vi "数据导入工具-main.vi"() -> ()   [LabVIEW 2016]
uses:
  <vilib>/Utility/sysdir.llb/System Directory Type.ctl
  <vilib>/addons/database/Connection.llb/DB Tools Open Connec (String).vi
  <userlib>/_LVST/sqlite_api/Core/Tables/SQLite_List Tables.vi
  <vilib>/addons/database/NI_Database_API.lvlib
  Access/Access Lib.lvlib
panel:
  in  "Password":string
  in  "Sqlite加密":bool
  in  "Sqlite解密":bool
  out "selected path":path caption="所选路径"
  in  "导入日志":string
  in  "导入SQLite":bool
  in  "ACCESS数据表":bool
  in  "列表框":i32[](listbox)
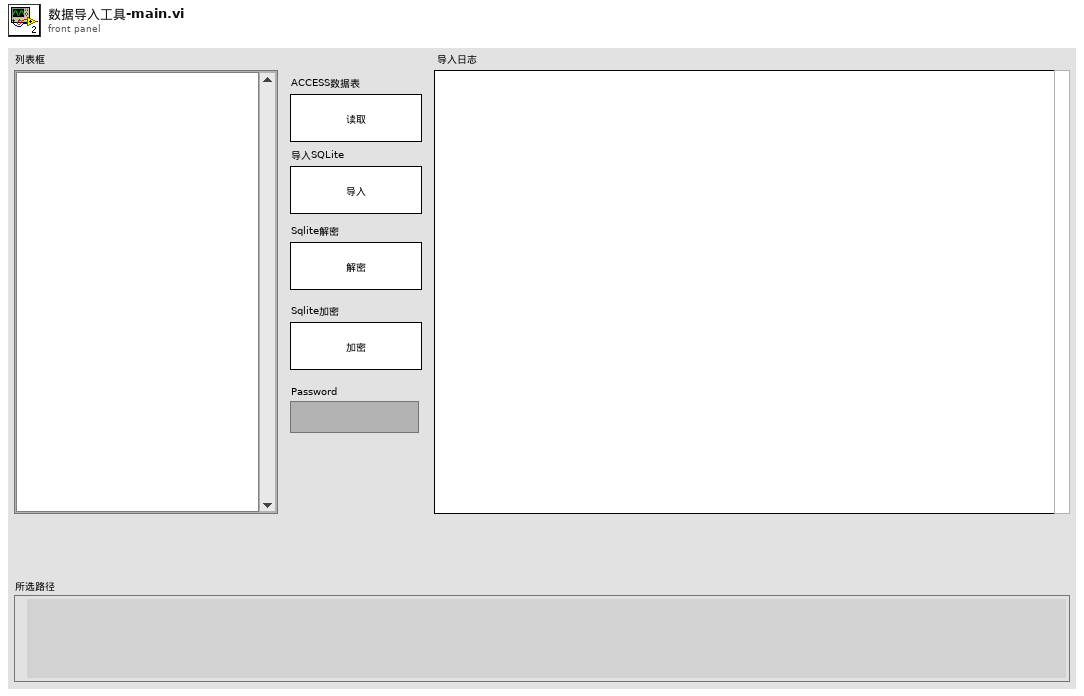
[diagram p1: front panel]
types:
  T1 = typedef "System Directory Type.ctl" = i32
  T2 = typedef "NI_Database_API.lvlib/Conn ObjectReference.ctl" = refnum<k1>
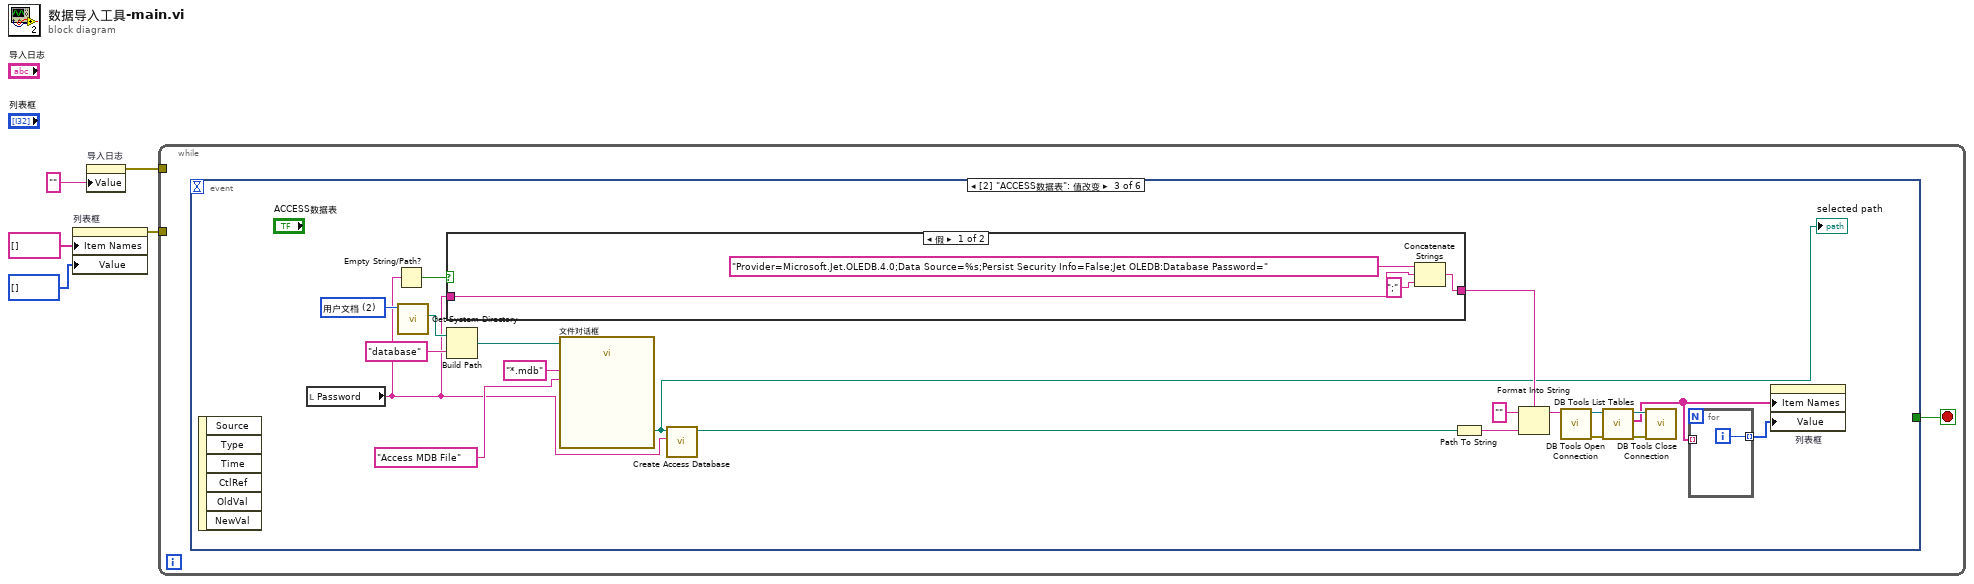
[diagram p0: block diagram]
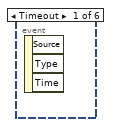
[diagram p2: hidden frame]
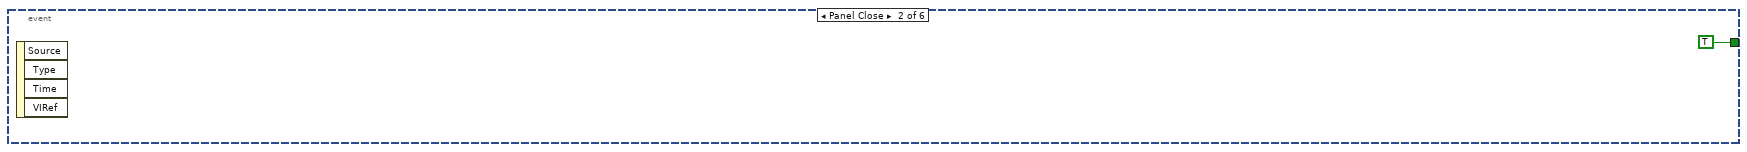
[diagram p3: hidden frame]
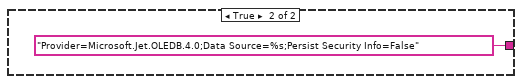
[diagram p4: hidden frame]
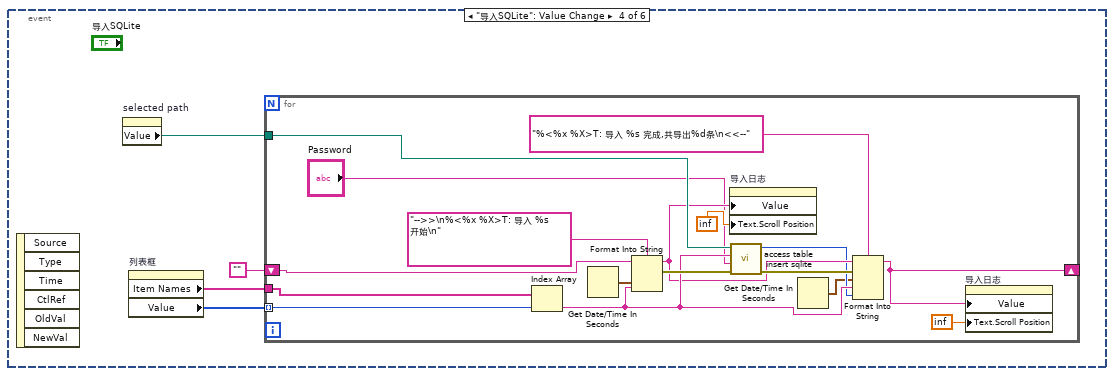
[diagram p5: hidden frame]
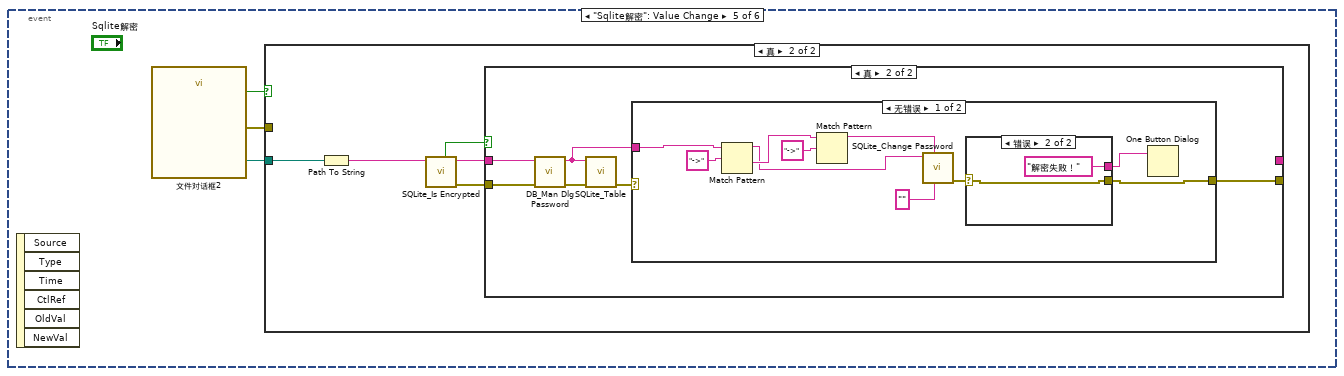
[diagram p6: hidden frame]
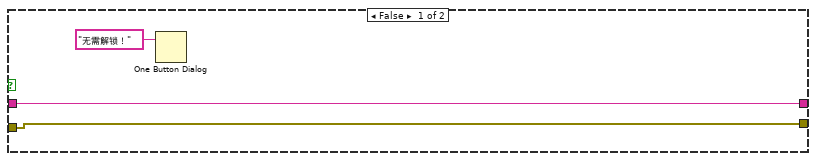
[diagram p8: hidden frame]
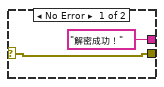
[diagram p9: hidden frame]
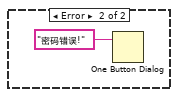
[diagram p10: hidden frame]
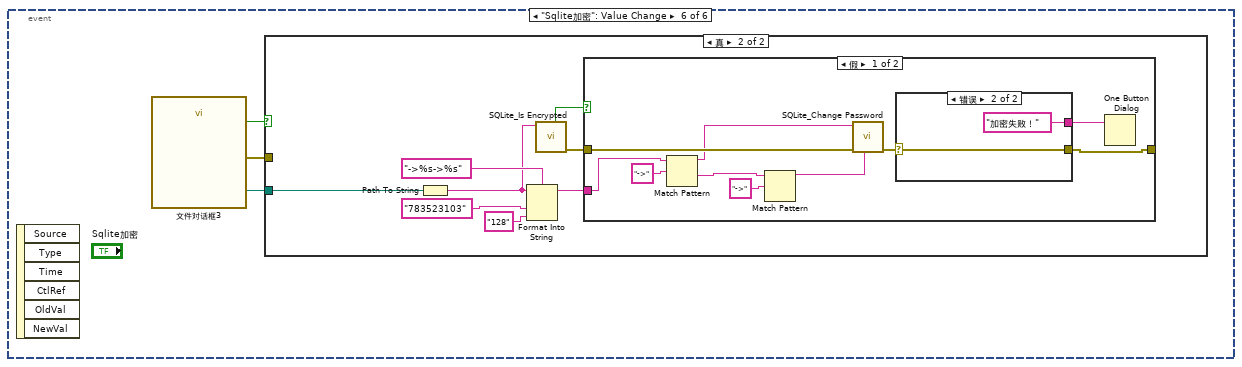
[diagram p11: hidden frame]
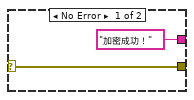
[diagram p13: hidden frame]
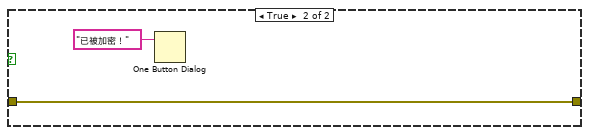
[diagram p14: hidden frame]
diagram:
  n1 = property on="列表框" class="LstBox (严格)"("Item Names"=string[] [] ("项名"), "Value"=i32[] [] ("列表框")) -> (error out=w3:errorcluster)  [unwired: 2 in, 1 out]
  n2 = property on="导入日志" class="Str"("Value"="" ("导入日志")) -> (error out=w1:errorcluster)  [unwired: 2 in, 1 out]
  n3 = while {
    tunnel: w3 -> [_]
    tunnel: w1 -> [_]
    stop <- w6 stop-if-true
    n4 = event shown="[2] \"ACCESS数据表\": 值改变" {
      selector: _ -> [_ _ _ _ _ _]
      dyn-events: _ -> [_ _ _ _ _ _]
      timeout: _ -> [_ _ _ _ _ _]
      tunnel: [_ TRUE _ _ _ _] -> w6
      event Timeout {
        n5 = event-data() -> ()  [unwired: 1 in, 3 out]
      }
      event Panel Close {
        n6 = event-data() -> ()  [unwired: 1 in, 4 out]
      }
      event "ACCESS数据表": Value Change {
        w27 = T1 2 items=["用户目录"=0, "用户桌面"=1, "用户文档"=2, "用户应用程序数据"=3, "用户设置"=4, "用户临时目录"=5, "公共文档"=6, "公共应用程序数据"=7, "公共设置"=8, "公共缓存"=13, "系统核心库"=9, "系统安装库"=10, "应用程序文件"=11, "启动盘根目录"=12] ("system directory type")
        n7 = event-data() -> ()  [unwired: 1 in, 6 out]
        n8 = local read "Password"() -> (w15:string)
        n9 = Empty String/Path?(string/path=w15) -> (empty?=w10:bool)
        n10 = call <vilib>:"Get System Directory.vi"("system directory type"=w27) -> ("system directory"=w26:path)  [unwired: 10 in]
        n11 = case shown="假" w10 {
          tunnel: [w28 "Provider=Microsoft.Jet.OLEDB.4.0;Data Source=%s;Persist Security Info=False" ("格式字符串")] -> w11
          tunnel: w15 -> [w31 _]
          frame False {
            n12 = Concatenate Strings("Provider=Microsoft.Jet.OLEDB.4.0;Data Source=%s;Persist Security Info=False;Jet OLEDB:Database Password=" ("格式字符串"), w31, ";" ("字符串")) -> (w28:string)
          }
          frame True {
          }
        }
        n13 = Build Path(base path=w26, name or relative path="database" ("名称或相对路径")) -> (appended path=w25:path)
        n14 = call "文件对话框"("start path"=w25, "pattern (all files)"="*.mdb", "pattern label"="Access MDB File") -> ("selected path"=w9:path)  [unwired: 9 in, 3 out]
        "selected path" <- w9
        n15 = call "Create Access Database.vi"("Password"=w15, "路径"=w9) -> ("路径 out"=w14:path)  [unwired: 8 in, 1 out]
        n16 = Path To String(path=w14) -> (string=w13:string)
        n17 = Format Into String(format string=w11, initial string="" ("初始字符串"), w13) -> (resulting string=w8:string)  [unwired: 1 in, 1 out]
        n18 = call-poly <vilib>:"DB Tools Open Connection.vi"("connection information"=w8) -> ("error out"=w21:errorcluster, "connection reference"=w20:T2)  [unwired: 7 in]
        n19 = call <vilib>:"DB Tools List Tables.vi"("error in (no error)"=w21, "connection reference"=w20) -> ("error out"=w18:errorcluster, "tables"=w17:string[], "connection reference out"=w19:T2)  [unwired: 3 in]
        n20 = call <vilib>:"DB Tools Close Connection.vi"("error in (no error)"=w18, "connection reference"=w19) -> ()  [unwired: 5 in, 1 out]
        n21 = for {
          tunnel: w17 -> [_] mode=indexing
          tunnel: [w33] -> w16 mode=indexing
          i -> [w33]
        }
        n22 = property on="列表框" class="LstBox (严格)"("Item Names"=w17, "Value"=w16) -> ()  [unwired: 2 in, 2 out]
      }
      event "导入SQLite": Value Change {
        n23 = event-data() -> ()  [unwired: 1 in, 6 out]
        n24 = property on="selected path" class="Path"() -> ("Value"=w37:path)  [unwired: 2 in, 2 out]
        n25 = property on="列表框" class="LstBox (严格)"() -> ("Item Names"=w35:string[], "Value"=w36:i32[])  [unwired: 2 in, 2 out]
        n26 = for {
          tunnel: w35 -> [w54]
          tunnel: w36 -> [w53] mode=indexing
          tunnel: w37 -> [w52]
          shift-right: [w46] -> _
          shift-left: "" -> [w51]
          n27 = Index Array(array=w54, index=w53) -> (element=w48:string)
          n28 = Get Date/Time In Seconds() -> (seconds since 1Jan1904=w43:timestamp)
          n29 = Format Into String(format string="-->>\n%<%x %X>T: 导入 %s 开始\n" ("格式字符串"), initial string=w51, w43, w48) -> (resulting string=w47:string, error out=w50:errorcluster)  [unwired: 1 in]
          n30 = property on="导入日志" class="Str"("Value"=w47, "Text.Scroll Position"=inf) -> ()  [unwired: 2 in, 2 out]
          n31 = call "access table insert sqlite.vi"("error in (no error)"=w50, "Password"="Password", "table"=w48, "路径"=w52) -> ("错误输出"=w49:errorcluster, "条数"=w45:i32)  [unwired: 6 in]
          n32 = Get Date/Time In Seconds() -> (seconds since 1Jan1904=w40:timestamp)
          n33 = Format Into String(format string="%<%x %X>T: 导入 %s 完成,共导出%d条\n<<--" ("格式字符串"), initial string=w47, error in=w49, w40, w48, w45) -> (resulting string=w46:string)  [unwired: 1 out]
          n34 = property on="导入日志" class="Str"("Value"=w46, "Text.Scroll Position"=inf) -> ()  [unwired: 2 in, 2 out]
        }
      }
      event "Sqlite解密": Value Change {
        n35 = event-data() -> ()  [unwired: 1 in, 6 out]
        n36 = call "文件对话框2"() -> ("selected path"=w57:path, "exists"=w55:bool, "error out"=w56:errorcluster)  [unwired: 12 in, 1 out]
        n37 = case shown="真" w55 {
          tunnel: w57 -> [_ w62]
          tunnel: w56 -> [_ _]
          frame False {
          }
          frame True {
            n38 = Path To String(path=w62) -> (string=w58:string)
            n39 = call <userlib>:"SQLite_Is Encrypted.vi"("Path"=w58) -> ("error out"=w61:errorcluster, "Path Out"=w60:string, "Encrypted?"=w59:bool)  [unwired: 7 in]
            n40 = case shown="真" w59 {
              tunnel: [w64 w69] -> _
              tunnel: w61 -> [w64 w71]
              tunnel: w60 -> [w65 w70]
              tunnel: [w65 _] -> _
              frame False {
                n41 = One Button Dialog(message="无需解锁！" ("消息")) -> ()  [unwired: 1 in, 1 out]
              }
              frame True {
                n42 = call <userlib>:"DB_Man Dlg Password.vi"("error in (no error)"=w71, "Path in"=w70) -> ("error out"=w67:errorcluster, "Path Out"=w68:string)  [unwired: 8 in]
                n43 = call-poly <userlib>:"SQLite_Table.vi"("DB Path"=w68, "error in (no error)"=w67) -> ("error out"=w66:errorcluster)  [unwired: 6 in, 2 out]
                n44 = case shown="无错误" w66 {
                  tunnel: [w74 _] -> w69
                  tunnel: w68 -> [w73 _]
                  frame No Error {
                    n45 = Match Pattern(string=w73, regular expression="->" ("正则表达式")) -> (before substring=w72:string, after substring=w77:string)  [unwired: 1 in, 2 out]
                    n46 = Match Pattern(string=w77, regular expression="->" ("正则表达式")) -> (before substring=w75:string)  [unwired: 1 in, 3 out]
                    n47 = call <userlib>:"SQLite_Change Password.vi"("New Password (Empty to remove)"="", "Old Password"=w75, "DB Path"=w72) -> ("error out"=w79:errorcluster)  [unwired: 7 in, 1 out]
                    n48 = case shown="错误" w79 {
                      selector: w79 -> [w82 w84]
                      tunnel: ["解密成功！" ("Old Password") "解密失败！" ("Old Password")] -> w81
                      tunnel: [w82 w84] -> w74
                      frame No Error {
                      }
                      frame Error {
                      }
                    }
                    n49 = One Button Dialog(message=w81) -> ()  [unwired: 1 in, 1 out]
                  }
                  frame Error {
                    n50 = One Button Dialog(message="密码错误!" ("消息")) -> ()  [unwired: 1 in, 1 out]
                  }
                }
              }
            }
          }
        }
      }
      event "Sqlite加密": Value Change {
        n51 = event-data() -> ()  [unwired: 1 in, 6 out]
        n52 = call "文件对话框3"() -> ("selected path"=w89:path, "exists"=w87:bool, "error out"=w88:errorcluster)  [unwired: 12 in, 1 out]
        n53 = case shown="真" w87 {
          tunnel: w89 -> [_ w97]
          tunnel: w88 -> [_ _]
          frame False {
          }
          frame True {
            n54 = Path To String(path=w97) -> (string=w91:string)
            n55 = Format Into String(format string="->%s->%s", initial string=w91, "783523103" ("Enter Password"), "128" ("Enter Password")) -> (resulting string=w90:string)  [unwired: 1 in, 1 out]
            n56 = call <userlib>:"SQLite_Is Encrypted.vi"("Path"=w91) -> ("error out"=w96:errorcluster, "Encrypted?"=w95:bool)  [unwired: 7 in, 1 out]
            n57 = case shown="假" w95 {
              tunnel: [w107 w113] -> _
              tunnel: w96 -> [w104 w113]
              tunnel: w90 -> [w102 _]
              frame False {
                n58 = Match Pattern(string=w102, regular expression="->" ("正则表达式")) -> (before substring=w101:string, after substring=w99:string)  [unwired: 1 in, 2 out]
                n59 = Match Pattern(string=w99, regular expression="->" ("正则表达式")) -> (before substring=w98:string)  [unwired: 1 in, 3 out]
                n60 = call <userlib>:"SQLite_Change Password.vi"("New Password (Empty to remove)"=w98, "error in (no error)"=w104, "DB Path"=w101) -> ("error out"=w105:errorcluster)  [unwired: 7 in, 1 out]
                n61 = case shown="错误" w105 {
                  selector: w105 -> [w108 w110]
                  tunnel: ["加密成功！" ("Old Password") "加密失败！" ("Old Password")] -> w106
                  tunnel: [w108 w110] -> w107
                  frame No Error {
                  }
                  frame Error {
                  }
                }
                n62 = One Button Dialog(message=w106) -> ()  [unwired: 1 in, 1 out]
              }
              frame True {
                n63 = One Button Dialog(message="已被加密！" ("消息")) -> ()  [unwired: 1 in, 1 out]
              }
            }
          }
        }
      }
    }
  }
